vi "SetAttributeViBoolean_SA-Marker_Source.vi"(7 "AttributeValue (Off)":bool, 8 "error in (no error)":errorcluster {"code" format="%.0x"}, 9 "AttributeID":u32(ring)=1150703 items=["SA_MARKER_CONTINUOUS_PEAK_SEARCH_ENABLED"=1150703, "SA_MARKER_COUPLE_ENABLED"=1150689, "SA_MARKER_ENABLED"=1150691, "SA_MARKER_FREQUENCYCOUNTER_GATE_TIME_AUTO_ENABLED"=1150684, "SA_MARKER_FREQUENCYCOUNTER_RESOLUTION_AUTO_ENABLED"=1150685, "SA_MARKER_FUNCTION_BAND_SPAN_AUTO_ENABLED"=1150704, "SA_MARKER_LINES_ENABLED"=1150696, "SA_MARKER_MEASUREATMARKER_COUPLE_ENABLED"=1150753, "SA_MARKER_MEASUREATMARKER_PRESELECTOR_CENTERING_ENABLED"=1150755, "SA_MARKER_NDBPOINTS_ENABLED"=1150686, "SA_MARKER_PEAK_EXCURSION_ENABLED"=1150706, "SA_MARKER_PEAK_TABLE_ENABLED"=1150697, "SA_MARKER_SIGNAL_TRACK_ENABLED"=1150718, "SA_MARKER_TABLE_ENABLED"=1150700, "SA_MARKER_THRESHOLD_ENABLED"=1150705, "SA_MARKER_TRACE_AUTO_ENABLED"=1150701, "SA_MARKER_X_AXIS_SCALE_AUTO_ENABLED"=1150699, "SA_SOURCE_FREQUENCY_OFFSET_ENABLED"=1150798, "SA_SOURCE_FREQUENCY_SWEEP_REVERSE_ENABLED"=1150796, "SA_SOURCE_LEVEL_AMPLITUDE_STEP_AUTO_ENABLED"=1150792, "SA_SOURCE_LEVEL_POWER_SWEEP_ENABLED"=1150789, "SA_SOURCE_RF_OUTPUT_ENABLED"=1150784], 11 "instrument handle":refnum<k15>) -> (0 "error out":errorcluster {"code" format="%.0x"}, 3 "instrument handle out":refnum<k15>)   [LabVIEW 2009, in "Keysight XSAn.lvlib"]
doc: "Sets a Boolean attribute from the instrument driver.\nThe following Attributes are supported:\n\nSA_MARKER_CONTINUOUS_PEAK_SEARCH_ENABLED\nSA_MARKER_COUPLE_ENABLED\nSA_MARKER_ENABLED\nSA_MARKER_FREQUENCYCOUNTER_GATE_TIME_AUTO_ENABLED\nSA_MARKER_FREQUENCYCOUNTER_RESOLUTION_AUTO_ENABLED\nSA_MARKER_FUNCTION_BAND_SPAN_AUTO_ENABLED\nSA_MARKER_LINES_ENABLED\nSA_MARKER_MEASUREATMARKER_COUPLE_ENABLED\nSA_MARKER_MEASUREATMARKER_PRESELECTOR_CENTERING_ENABLED\nSA_MARKER_NDBPOINTS_ENABLED\nSA_MARKER_PEAK_EXCURSION_ENABLED\nSA_MARKER_PEAK_TABLE_ENABLED\nSA_MARKER_SIGNAL_TRACK_ENABLED\nSA_MARKER_TABLE_ENABLED\nSA_MARKER_THRESHOLD_ENABLED\nSA_MARKER_TRACE_AUTO_ENABLED\nSA_MARKER_X_AXIS_SCALE_AUTO_ENABLED\nSA_SOURCE_FREQUENCY_OFFSET_ENABLED\nSA_SOURCE_FREQUENCY_SWEEP_REVERSE_ENABLED\nSA_SOURCE_LEVEL_AMPLITUDE_STEP_AUTO_ENABLED\nSA_SOURCE_LEVEL_POWER_SWEEP_ENABLED\nSA_SOURCE_RF_OUTPUT_ENABLED"
uses:
  <instrlib>/Keysight XSAn/Keysight XSAn.lvlib
  AgXSAn.dll
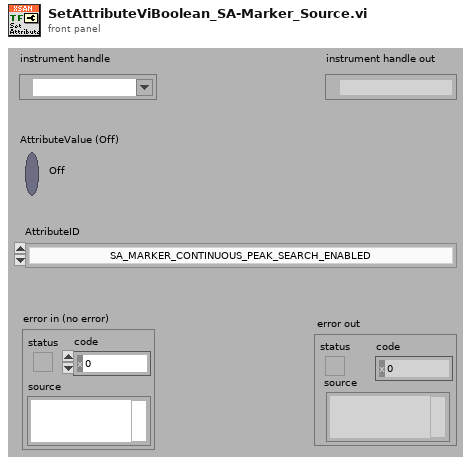
[diagram p1: front panel]
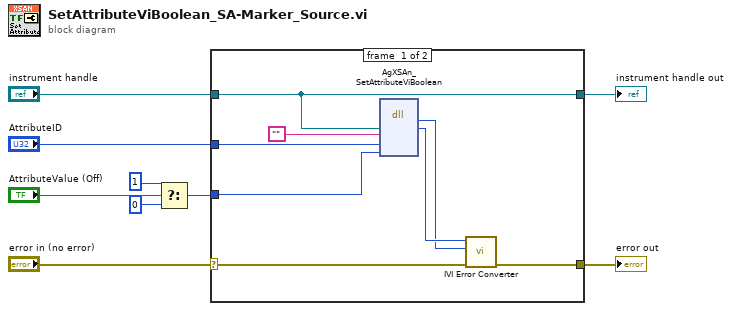
[diagram p0: block diagram]
diagram:
  n1 = Select(t=u16 1, s="AttributeValue (Off)", f=u16 0) -> (s? t:f=w2:u16)
  n2 = case shown="No Error" "error in (no error)" {
    selector: "error in (no error)" -> [w15 w19]
    tunnel: [w14 w19] -> w9
    tunnel: "instrument handle" -> [w11 w18]
    tunnel: "AttributeID" -> [w13 _]
    tunnel: w2 -> [w12 _]
    tunnel: [w11 w18] -> w1
    frame #0 {
      n3 = dll-call lib="AgXSAn**.dll" fn="AgXSAn_SetAttributeViBoolean"("Vi"=w11, "RepCapIdentifier"="", "AttributeID"=w13, "AttributeValue"=w12) -> ("return type"=w16:i32, "Vi"=w17:u32)  [unwired: 6 in, 2 out]
      n4 = call <instrlib>:"IVI Error Converter.vi"("error in (no error)"=w15, "IVI error code (0)"=w16, "instrument handle"=w17) -> ("error out"=w14:errorcluster)  [unwired: 7 in, 1 out]
    }
    frame #1 {
    }
  }
  "error out" <- w9
  "instrument handle out" <- w1
